vi "Self-Test.vi"(8 "error in (no error)":errorcluster, 11 "PicoScope 3000a in":refnum<class "PicoScope 3000a.lvclass">) -> (0 "error out":errorcluster, 2 "Self-Test Passed? (T:Yes)":bool, 3 "PicoScope 3000a out":refnum<class "PicoScope 3000a.lvclass">)   [LabVIEW 2018, in "PicoScope 3000a.lvlib" / "PicoScope 3000a.lvclass"]
doc: "This Override method is used to call the Self-Test function of the Oscope instrument. The boolean output 'Self-Test Passed? (T:Yes)' carries out the Self-Test result."
uses:
  PicoScope 3000a.lvclass
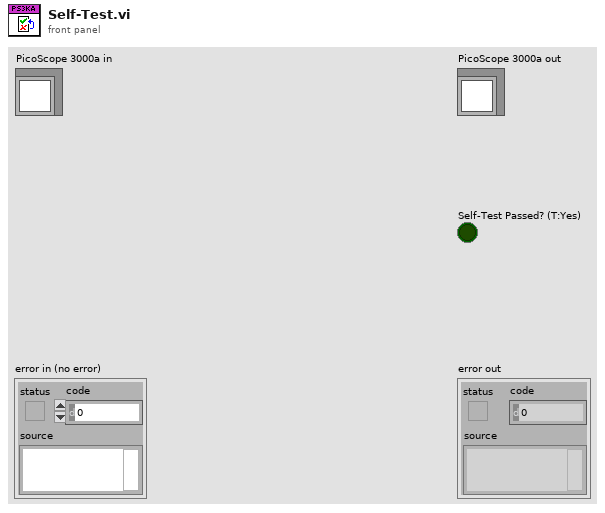
[diagram p1: front panel]
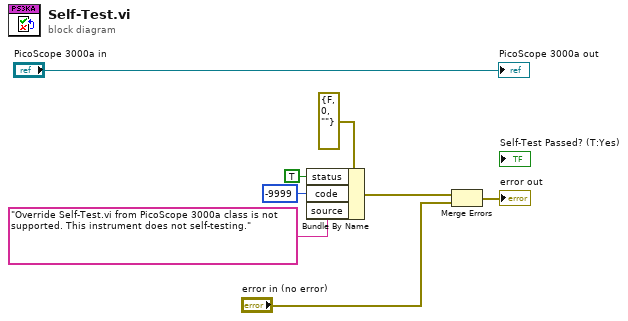
[diagram p0: block diagram]
diagram:
  n1 = Bundle By Name(cluster=errorcluster {"status"=FALSE, "code"=0, "source"=""} ("error constant"), "status"=TRUE, "code"=-9999, "source"="Override Self-Test.vi from PicoScope 3000a class is not supported. This instrument does not self-testing.") -> (w4:errorcluster)
  n2 = Merge Errors(w4, "error in (no error)") -> (→"error out":errorcluster)
  "PicoScope 3000a out" <- "PicoScope 3000a in"
